vi "Configure Modulation Low Level (FSK Rate).vi"(8 "error in (no error)":errorcluster, 10 "Shift Rate (10 Hz)":dbl=10.0, 11 "VISA resource name":refnum<visa-resource-name>) -> (0 "error out":errorcluster, 3 "VISA resource name out":refnum<visa-resource-name>)   [LabVIEW 2017, in "Keithley 3390.lvlib"]
doc: "Sets the rate for the frequency shift keying modulation technique. FSK Rate is the rate at which the output frequency shifts between the carrier and the hop frequency when the internal source is selected."
uses:
  Keithley 3390.lvlib
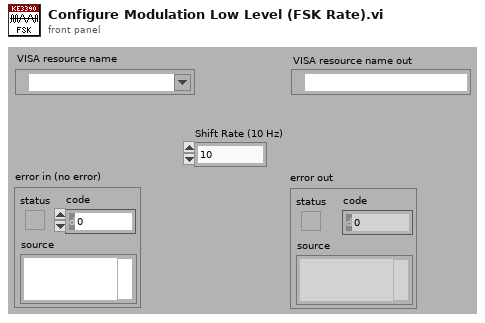
[diagram p1: front panel]
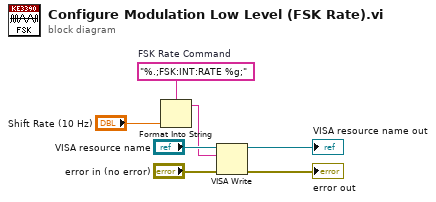
[diagram p0: block diagram]
diagram:
  w4 = "%.;FSK:INT:RATE %g;"  # FSK Rate Command
  n1 = Format Into String(format string=w4, "Shift Rate (10 Hz)") -> (resulting string=w5:string)  [unwired: 2 in, 1 out]
  n2 = VISA Write(VISA resource name="VISA resource name", write buffer=w5, error in (no error)="error in (no error)") -> (VISA resource name out=→"VISA resource name out":refnum<visa-resource-name>, error out=→"error out":errorcluster)  [unwired: 1 out]
